vi "作为主程序使用.vi"() -> ()   [LabVIEW 2017]
panel:
  out "数值 3":dbl
  in  "数值 2":dbl
  in  "数值":dbl
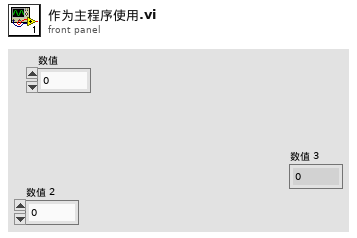
[diagram p1: front panel]
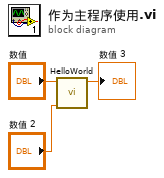
[diagram p0: block diagram]
diagram:
  n1 = call "HelloWorld.vi"("数值 2"="数值 2", "数值"="数值") -> ("数值 3"=→"数值 3":dbl)  [unwired: 9 in]
